vi "VerifyMeasurementsDirectory.vi"(7 "Key Found?":bool, 10 "Error in":errorcluster, 11 "Measurements Directory Path in":path) -> (2 "Error out":errorcluster, 3 "Measurements Directory Path out":path)   [LabVIEW 2019]
uses:
  <vilib>/Utility/sysdir.llb/System Directory Type.ctl
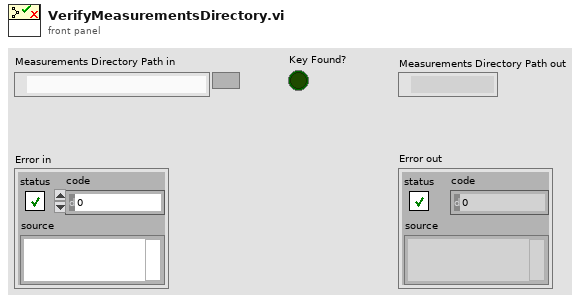
[diagram p1: front panel]
types:
  T1 = typedef "System Directory Type.ctl" = i32
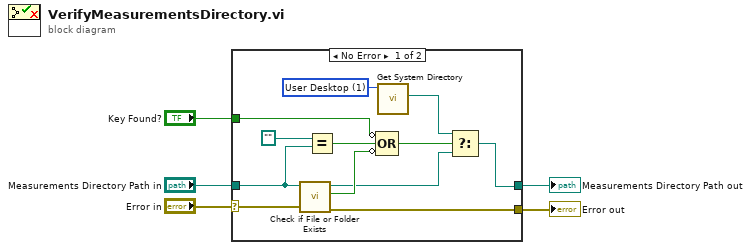
[diagram p0: block diagram]
diagram:
  n1 = case shown="No Error" "Error in" {
    selector: "Error in" -> [w7 w19]
    tunnel: "Measurements Directory Path in" -> [w17 w18]
    tunnel: [w9 w18] -> w4
    tunnel: [w8 w19] -> w3
    tunnel: "Key Found?" -> [w6 _]
    frame No Error {
      w11 = T1 1 items=["User Home"=0, "User Desktop"=1, "User Documents"=2, "User Application Data"=3, "User Preferences"=4, "User Temporary"=5, "Public Documents"=6, "Public Application Data"=7, "Public Preferences"=8, "Public Cache"=13, "System Core Libraries"=9, "System Installed Libraries"=10, "Application Files"=11, "Boot Volume Root"=12] ("system directory type")
      n2 = call <vilib>:"Check if File or Folder Exists.vi"("error in (no error)"=w7, "path"=w17) -> ("error out"=w8:errorcluster, "file or folder exists?"=w14:bool, "dup path"=w12:path)  [unwired: 7 in]
      n3 = Equal?(x=path "", y=w17) -> (x = y?=w15:bool)
      n4 = Compound Arithmetic op=OR(invert w6, w15, invert w14) -> (w13:bool)
      n5 = call <vilib>:"Get System Directory.vi"("system directory type"=w11) -> ("system directory"=w10:path)  [unwired: 10 in]
      n6 = Select(t=w10, s=w13, f=w12) -> (s? t:f=w9:path)
    }
    frame Error {
    }
  }
  "Measurements Directory Path out" <- w4
  "Error out" <- w3
